vi "SSC Relay Control Single Action Per-Relay Pin.vi"(0 "SSC Relay in":T1[](array[typedef]), 1 "Wait Between Relays (s)":dbl, 5 "Relay Action":T3=21 items=["Open Relay"=20, "Close Relay"=21], 7 "Settling Time (s)":dbl format="%#_12p", 9 "Relay Pins":string[](array[string]), 11 "error in":errorcluster) -> (4 "SSC Relay out":T1[](array[typedef]), 8 "Completed Relay Operations":T2[](array[typedef]) {"Desired State" items=["Open Relay"=20, "Close Relay"=21]}, 15 "error out":errorcluster)   [LabVIEW 2019]
doc: "Performs the specified relay action on all Relays configured in the SSC Relay session, one Relay at a time. The function will then wait a specified amount of time if the Settling Time (s) input is wired. \n\nUse the Wait Between Relays (s) input if a wait time is desired between relay actions."
uses:
  SSC Relay.ctl
  <instrlib>/niSwitch/niSwitch.llb/niSwitch Relay Action.ctl
  SubVIs/TSM Relay Completed Operations.ctl
  SSC Relay Control Core.vi
  Single SSC Relay NI-Switch Control.vi
  Single SSC Relay Fill Additional Error info.vi
  SSC Relay Expand Action Array to All Sessions.vi
  <vilib>/Utility/error.llb/Error Cluster From Error Code.vi
  <instrlib>/niSwitch/niSwitch.llb/niSwitch Get Relay Position.vi
  <instrlib>/niSwitch/niSwitch.llb/niSwitch Relay Control.vi
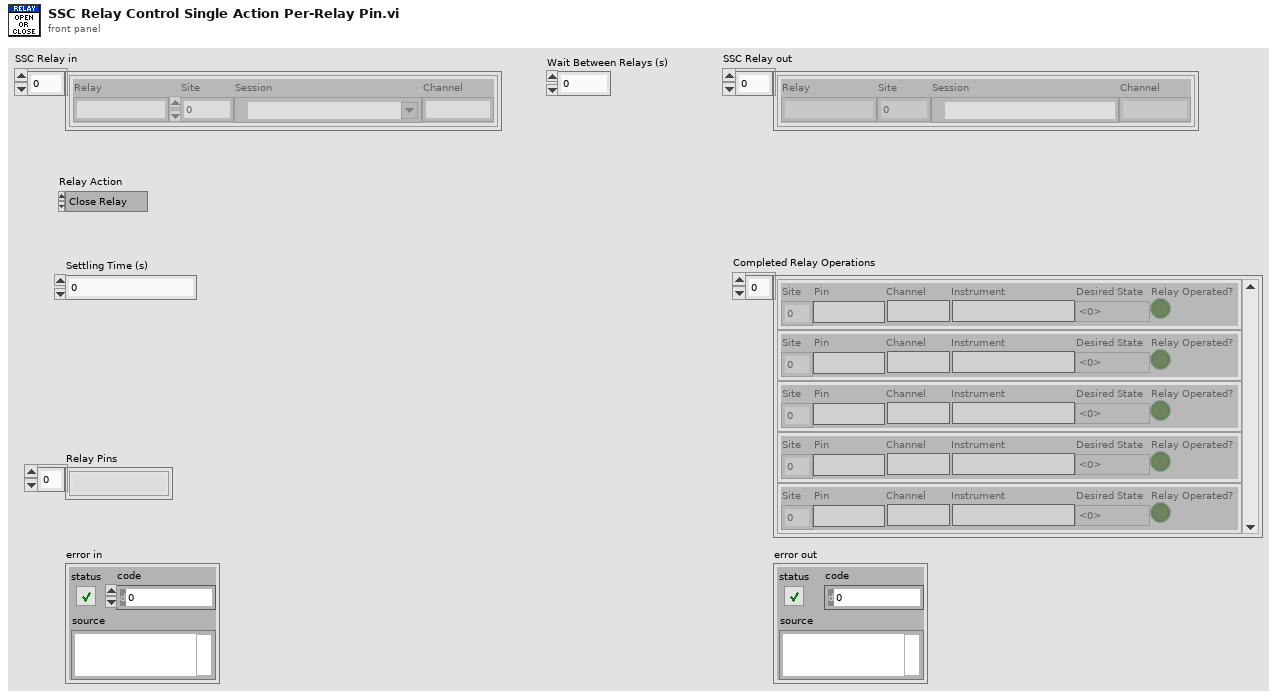
[diagram p1: front panel]
types:
  T1 = typedef "SSC Relay.ctl" = cluster{"Relay":string, "Site":i32, "Session":refnum<k15>, "Channel":string}
  T2 = typedef "TSM Relay Completed Operations.ctl" = cluster{"Site":i32, "Pin":string, "Channel":string, "Instrument":string, "Desired State":T3, "Relay Operated?":bool}
  T3 = typedef "niSwitch Relay Action.ctl" = i32
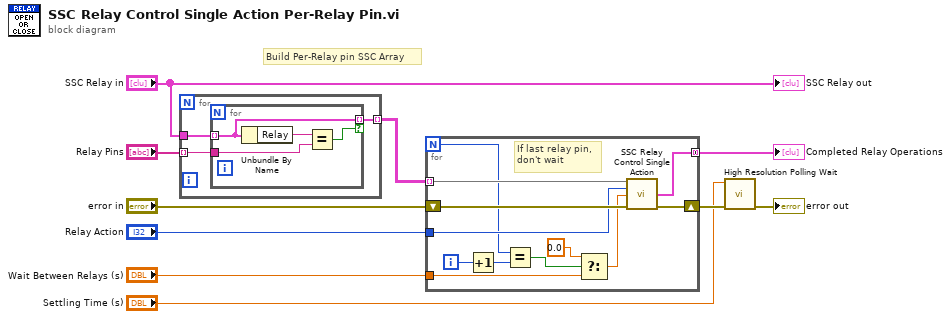
[diagram p0: block diagram]
diagram:
  # "Build Per-Relay pin SSC Array"
  n1 = for {
    tunnel: "SSC Relay in" -> [w13]
    tunnel: [w12] -> w10 mode=indexing
    tunnel: "Relay Pins" -> [w11] mode=indexing
    n2 = for {
      tunnel: w13 -> [w17] mode=indexing
      tunnel: [w17] -> w12 mode=indexing if=w15
      tunnel: w11 -> [w14]
      n3 = Unbundle By Name(w17) -> ("Relay"=w16:string)
      n4 = Equal?(x=w16, y=w14) -> (x = y?=w15:bool)
    }
  }
  n5 = for {
    N -> [w19]
    tunnel: "Wait Between Relays (s)" -> [w27]
    tunnel: w10 -> [w20] mode=indexing
    tunnel: [w18] -> w5 mode=concatenating
    tunnel: "Relay Action" -> [w21]
    shift-right: [w23] -> w3
    shift-left: "error in" -> [w24]
    i -> [w29]
    # "If last relay pin, don't wait"
    n6 = Increment(x=w29) -> (x+1=w25:i32)
    n7 = Equal?(x=w19, y=w25) -> (x = y?=w28:bool)
    n8 = Select(t=0.0, s=w28, f=w27) -> (s? t:f=w22:dbl)
    n9 = call "SSC Relay Control Single Action.vi"("SSC Relay in"=w20, "Relay Action"=w21, "Settling Time (s)"=w22, "error in"=w24) -> ("Completed Relay Operations"=w18:T2[], "error out"=w23:errorcluster)  [unwired: 9 in, 1 out]
  }
  "Completed Relay Operations" <- w5
  n10 = call <vilib>:"High Resolution Polling Wait.vi"("error in (no error)"=w3, "seconds to wait"="Settling Time (s)") -> ("error out"=→"error out":errorcluster)  [unwired: 9 in]
  "SSC Relay out" <- "SSC Relay in"
